vi "Inclino3D_final.vi"() -> ()   [LabVIEW 2022 SP3]
uses:
  <vilib>/picture/3D Picture Control/Object/Create Object (name).vi
  <vilib>/picture/3D Picture Control/NI_3D Picture Control.lvlib
panel:
  out "angle de tangage en rad 2":dbl
  out "z en g 2":dbl
  out "y en g 2":dbl
  out "x 2":dbl
  out "z 2":dbl
  out "y 2":dbl
  out "x en g 2":dbl
  out "3D Picture":refnum<vi>(3d-picture)
  out "Roulis (°)":i16(knob) scale=-90.0..90.0
  out "Tangage (°)":i16(knob) scale=-90.0..90.0
  in  "?":bool
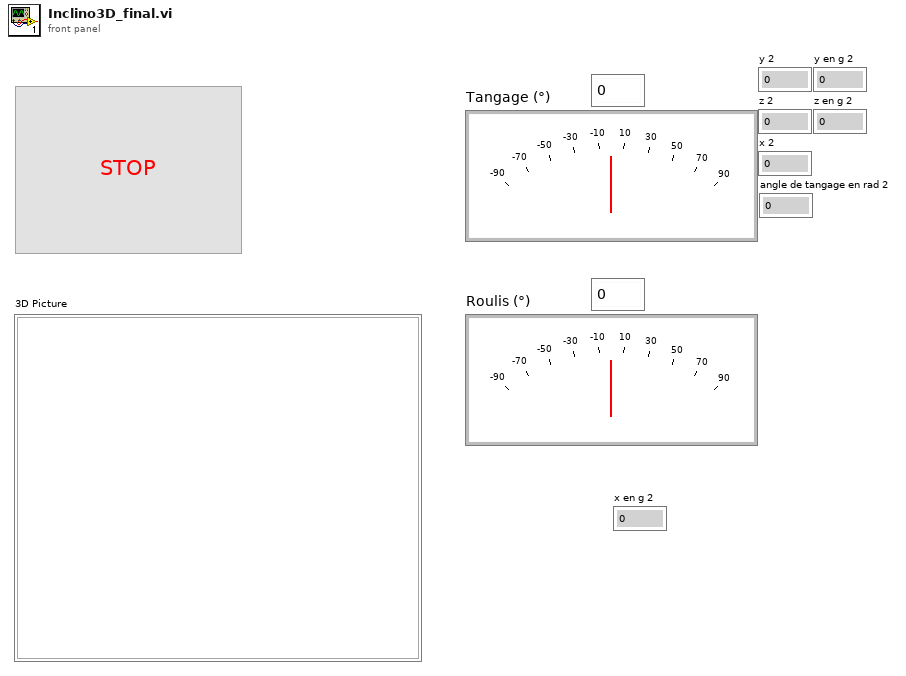
[diagram p1: front panel]
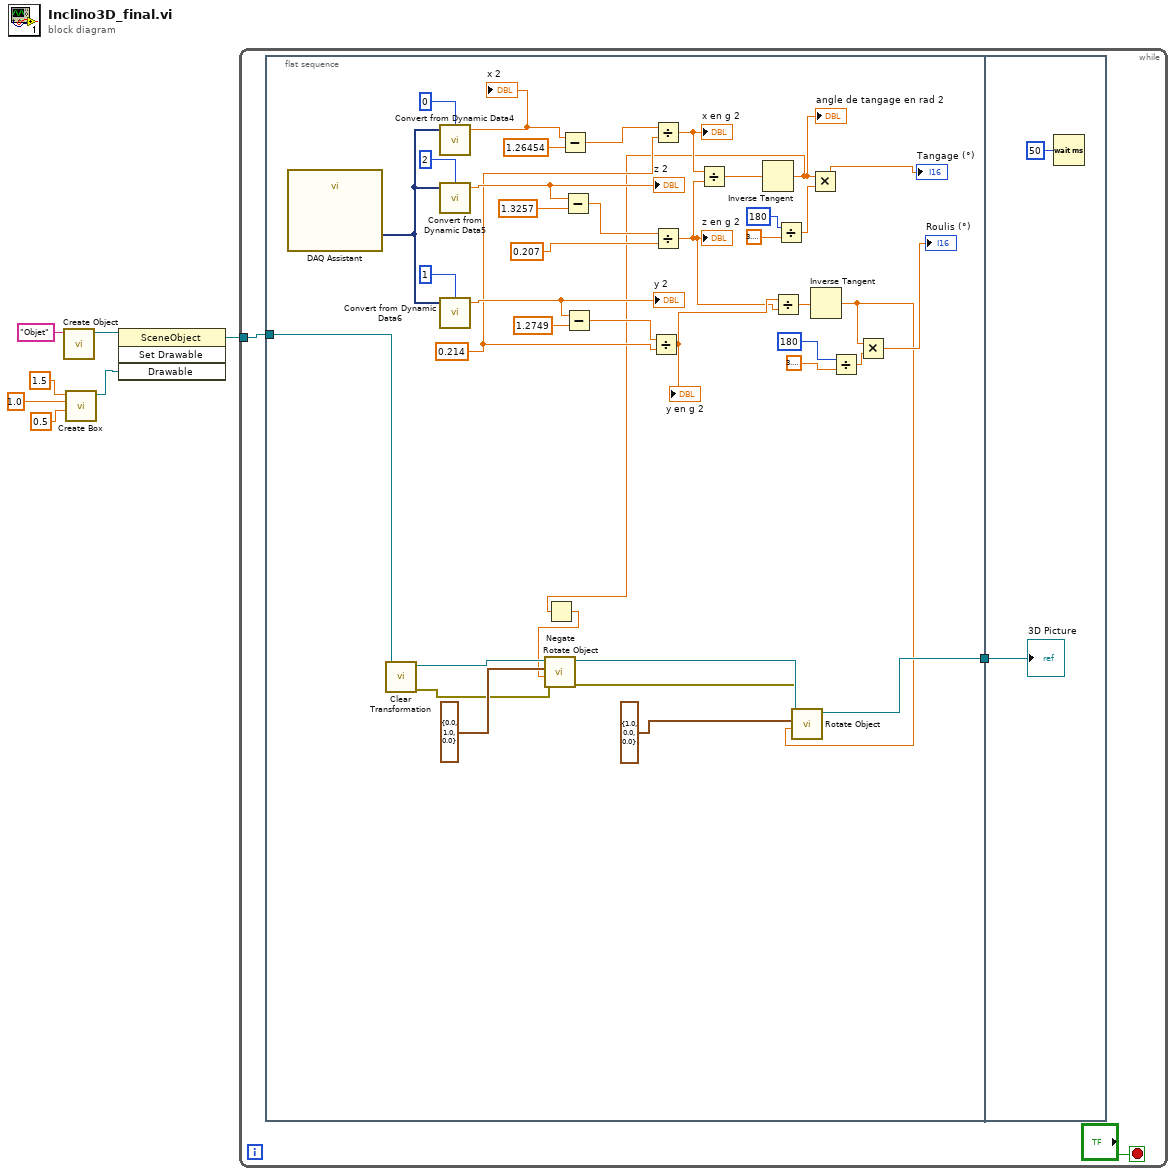
[diagram p0: block diagram]
diagram:
  n1 = call-poly <vilib>:"Create Object.vi"("Name"="Objet") -> ("Scene:New Object"=w3:refnum<vi>)  [unwired: 9 in, 1 out]
  n2 = call <vilib>:"Create Box.vi"("Length Z"=sgl 0.5, "Length Y"=sgl 1.0, "Length X"=sgl 1.5) -> ("New Box Refnum"=w2:refnum<vi>)  [unwired: 7 in, 1 out]
  n3 = invoke class="SceneObject" method="Set Drawable"(reference=w3, "Drawable"=w2) -> (reference out=w1:refnum<vi>)  [unwired: 2 in, 3 out]
  n4 = while {
    tunnel: w1 -> [w9]
    stop <- "?" stop-if-true
    n5 = flat-sequence {
      tunnel: w9 -> [w46]
      tunnel: [w42] -> w8
      tunnel: w8 -> [w50]
      frame #0 {
        w23 = 0.214
        n6 = call "DAQ Assistant"() -> ("data"=w24:dynamicdata)  [unwired: 17 in, 2 out]
        n7 = call <vilib>:"Clear Transformation.vi"("Object Refnum In"=w46) -> ("error out"=w47:errorcluster, "Object Refnum Out"=w49:refnum<vi>)  [unwired: 9 in]
        n8 = call "Convert from Dynamic Data4"("Dynamic Data Type"=w24, "Channel"=0) -> ("Scalar"=w38:dbl)  [unwired: 2 in]
        "x 2" <- w38
        n9 = call "Convert from Dynamic Data5"("Dynamic Data Type"=w24, "Channel"=2) -> ("Scalar"=w36:dbl)  [unwired: 2 in]
        "z 2" <- w36
        n10 = call "Convert from Dynamic Data6"("Dynamic Data Type"=w24, "Channel"=1) -> ("Scalar"=w34:dbl)  [unwired: 2 in]
        "y 2" <- w34
        n11 = Subtract(x=w38, y=1.26454) -> (x-y=w37:dbl)
        n12 = Subtract(x=w36, y=1.3257) -> (x-y=w35:dbl)
        n13 = Subtract(x=w34, y=1.2749) -> (x-y=w33:dbl)
        n14 = Divide(x=w33, y=w23) -> (x/y=w18:dbl)
        "y en g 2" <- w18
        n15 = Divide(x=w37, y=w23) -> (x/y=w41:dbl)
        "x en g 2" <- w41
        n16 = Divide(x=w35, y=0.207) -> (x/y=w17:dbl)
        "z en g 2" <- w17
        n17 = Divide(x=w41, y=w17) -> (x/y=w40:dbl)
        n18 = Inverse Tangent(1:w40) -> (0:w12:dbl)
        "angle de tangage en rad 2" <- w12
        n19 = Negate(x=w12) -> (-x=w13:dbl)
        n20 = call <vilib>:"Rotate Object.vi"("error in (no error)"=w47, "Angle"=w13, "Axis"=cluster{"X":sgl, "Y":sgl, "Z":sgl} {"X"=0.0, "Y"=1.0, "Z"=0.0}, "Scene.Object In"=w49) -> ("error out"=w44:errorcluster, "Scene.Object Out"=w45:refnum<vi>)  [unwired: 6 in]
        n21 = Divide(x=w18, y=w17) -> (x/y=w22:dbl)
        n22 = Divide(x=180, y=3.141592653589793) -> (x/y=w39:dbl)
        n23 = Multiply(x=w12, y=w39) -> (x*y=→"Tangage (°)":dbl)
        n24 = Inverse Tangent(1:w22) -> (0:w11:dbl)
        n25 = call <vilib>:"Rotate Object.vi"("error in (no error)"=w44, "Angle"=w11, "Axis"=cluster{"X":sgl, "Y":sgl, "Z":sgl} {"X"=1.0, "Y"=0.0, "Z"=0.0}, "Scene.Object In"=w45) -> ("Scene.Object Out"=w42:refnum<vi>)  [unwired: 6 in, 1 out]
        n26 = Divide(x=180, y=3.141592653589793) -> (x/y=w19:dbl)
        n27 = Multiply(x=w11, y=w19) -> (x*y=→"Roulis (°)":dbl)
      }
      frame #1 {
        n28 = Wait (ms)(milliseconds to wait=u32 50) -> ()  [unwired: 1 out]
        "3D Picture" <- w50
      }
    }
  }
